vi "Gview-MenuStructure.vi"() -> (1 "MenuStructure":T1=[{"After_tag"="", "MenuItems"=[{"name"="File", "tag"="File", "checked"=FALSE, "enabled"=TRUE}, {"name"="Autoscale", "tag"="Auto", "checked"=FALSE, "enabled"=TRUE}, {"name"="Timeline", "tag"="Time", "checked"=FALSE, "enabled"=TRUE}, {"name"="Preset", "tag"="Preset", "checked"=FALSE, "enabled"=TRUE}, {"name"="Y-Scale", "tag"="Yscale", "checked"=FALSE, "enabled"=TRUE}, {"name"="Options", "tag"="Options", "checked"=FALSE, "enabled"=TRUE}]}, {"After_tag"="File", "MenuItems"=[{"name"="Export image", "tag"="png", "checked"=FALSE, "enabled"=TRUE}, {"name"="Export Excel", "tag"="Excel", "checked"=FALSE, "enabled"=TRUE}, {"name"="app_separator", "tag"="app_separator", "checked"=FALSE, "enabled"=FALSE}, {"name"="Close Graph", "tag"="Exit", "checked"=FALSE, "enabled"=TRUE}, {"name"="Exit All Graphs", "tag"="ExitAll", "checked"=FALSE, "enabled"=TRUE}]}, {"After_tag"="Excel", "MenuItems"=[{"name"="Hi-resolution", "tag"="Excel-HI", "checked"=FALSE, "enabled"=TRUE}, {"name"="Samples shown", "tag"="Excel-Graph", "checked"=FALSE, "enabled"=TRUE}, {"name"="Low-Resolution", "tag"="Excel-Low", "checked"=FALSE, "enabled"=TRUE}]}, {"After_tag"="Options", "MenuItems"=[{"name"="Menu bar", "tag"="MenuBar", "checked"=TRUE, "enabled"=TRUE}, {"name"="Context menu", "tag"="MenuCtx", "checked"=FALSE, "enabled"=TRUE}, {"name"="Legend (L)", "tag"="Legend", "checked"=TRUE, "enabled"=TRUE}, {"name"="app_separator", "tag"="app_separator", "checked"=FALSE, "enabled"=FALSE}, {"name"="Toolbar", "tag"="ToolBar", "checked"=FALSE, "enabled"=TRUE}]}, {"After_tag"="Time", "MenuItems"=[{"name"="30 seconds", "tag"="T_30sec", "checked"=FALSE, "enabled"=TRUE}, {"name"="2 minutes", "tag"="T_2min", "checked"=FALSE, "enabled"=TRUE}, {"name"="10 minutes", "tag"="T_10min", "checked"=FALSE, "enabled"=TRUE}, {"name"="app_separator", "tag"="app_separator", "checked"=FALSE, "enabled"=TRUE}, {"name"="1 hour", "tag"="T_1hr", "checked"=FALSE, "enabled"=TRUE}, {"name"="4 hours", "tag"="T_4hr", "checked"=FALSE, "enabled"=TRUE}, {"name"="8 hours", "tag"="T_8hr", "checked"=FALSE, "enabled"=TRUE}, {"name"="app_separator", "tag"="app_separator", "checked"=FALSE, "enabled"=TRUE}, {"name"="Today", "tag"="T_Today", "checked"=FALSE, "enabled"=TRUE}, {"name"="1 days", "tag"="T_1day", "checked"=FALSE, "enabled"=TRUE}, {"name"="2 days", "tag"="T_2days", "checked"=FALSE, "enabled"=TRUE}, {"name"="5 days", "tag"="T_5days", "checked"=FALSE, "enabled"=TRUE}, {"name"="app_separator", "tag"="app_separator", "checked"=FALSE, "enabled"=TRUE}, {"name"="This week", "tag"="T_Week", "checked"=FALSE, "enabled"=TRUE}, {"name"="1 Week", "tag"="T_1wk", "checked"=FALSE, "enabled"=TRUE}, {"name"="2 Weeks", "tag"="T_2wks", "checked"=FALSE, "enabled"=TRUE}, {"name"="This month", "tag"="T_month", "checked"=FALSE, "enabled"=TRUE}, {"name"="1 Month", "tag"="T_1month", "checked"=FALSE, "enabled"=TRUE}, {"name"="app_separator", "tag"="app_separator", "checked"=FALSE, "enabled"=FALSE}, {"name"="3 months", "tag"="T_3months", "checked"=FALSE, "enabled"=TRUE}, {"name"="6 months", "tag"="T_6months", "checked"=FALSE, "enabled"=TRUE}, {"name"="One Year", "tag"="T_1year", "checked"=FALSE, "enabled"=TRUE}, {"name"="This Year", "tag"="T_Year", "checked"=FALSE, "enabled"=TRUE}]}, {"After_tag"="ToolBar", "MenuItems"=[{"name"="Native", "tag"="ToolNative", "checked"=FALSE, "enabled"=TRUE}, {"name"="Bare", "tag"="ToolBare", "checked"=FALSE, "enabled"=TRUE}, {"name"="Gradient", "tag"="ToolGradient", "checked"=FALSE, "enabled"=TRUE}]}])   [LabVIEW 2020, in "Gviewer.lvclass"]
doc: "Andre Koelewijn, 3 jan 2021, rev 0\n\nDefinition of Graph Menu structure\nThis defines the menu bar and the right click context menu appearance."
uses:
  Gviewer.lvclass
  MenuStructure.ctl
  C:/Users/Andre/Desktop/Menu/NEW/MenuItem.ctl
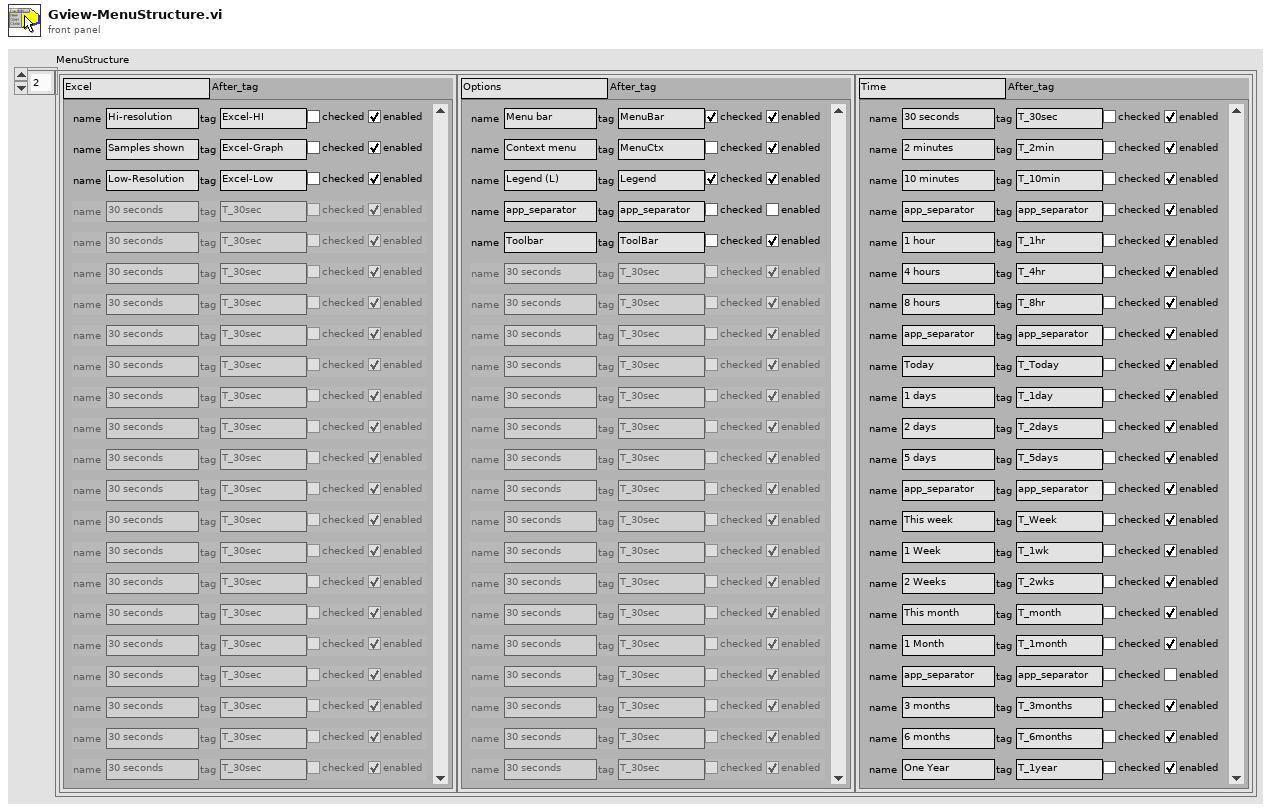
[diagram p1: front panel]
types:
  T1 = typedef "MenuStructure.ctl" = cluster{"After_tag":string, "MenuItems":T2[]}[]
  T2 = typedef "MenuItem.ctl" = cluster{"name":string, "tag":string, "checked":bool, "enabled":bool}
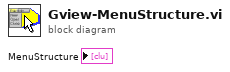
[diagram p0: block diagram]
diagram:
